vi "create s file from tdms of failed scan.vi"() -> ()   [LabVIEW 2020]
uses:
  Scan info_typdef.ctl
panel:
  in  "delete exising added channels":bool=TRUE
  out "TDMS path used":path
  out "appargs":string[](array[string])
  in  "append shot and bin #s":bool=TRUE
  out "device data Spreadsheet format":string[][](array[string])
  in  "TDMS path":path
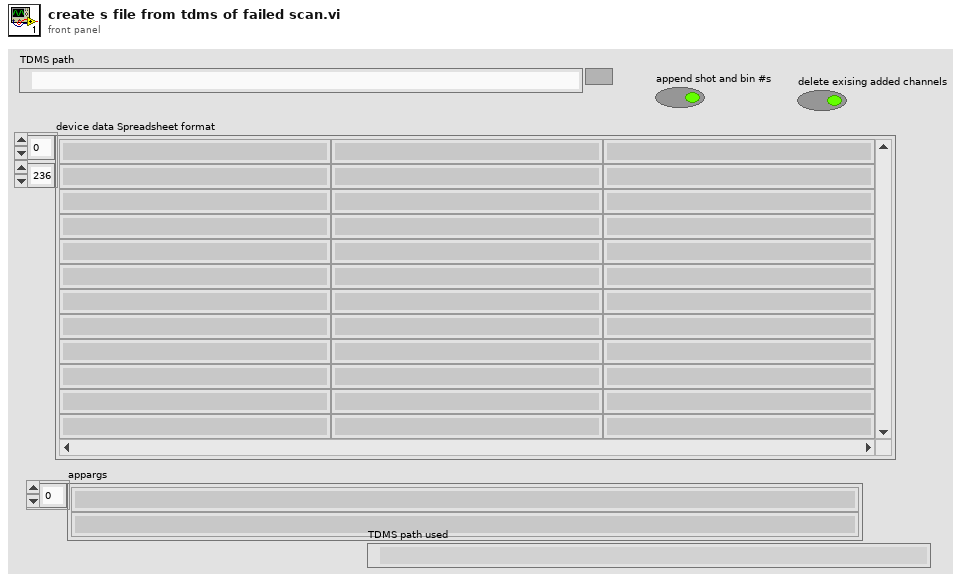
[diagram p1: front panel]
types:
  T1 = typedef "Scan info_typdef.ctl" = cluster{"# BG shots":i32, "Max Shot Number":i32, "Scan Number":i32}
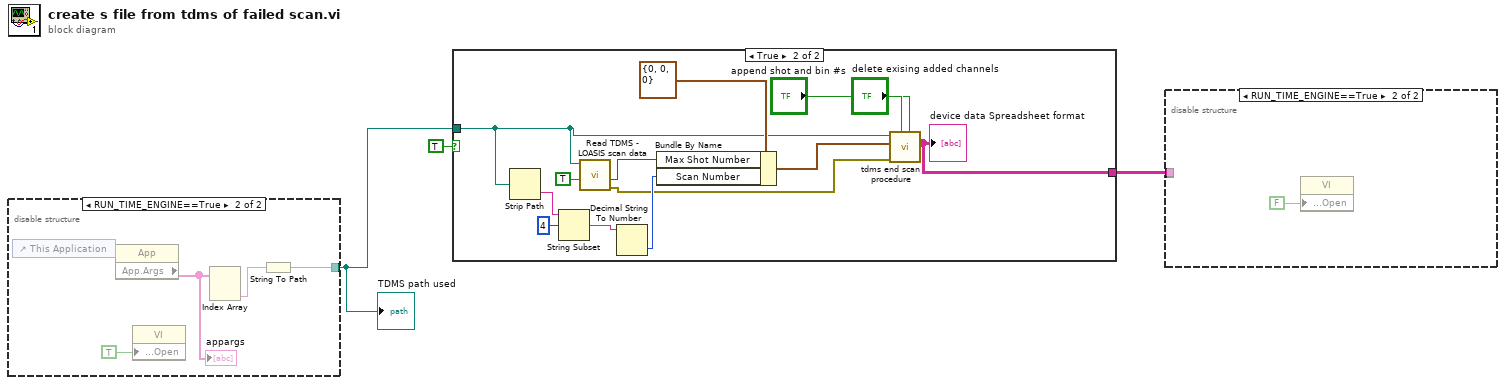
[diagram p0: block diagram]
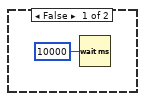
[diagram p3: hidden frame]
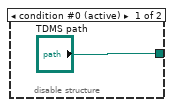
[diagram p4: hidden frame]
diagram:
  n1 = disable-structure shown="RUN_TIME_ENGINE==True" {
    disable-tunnel: ["TDMS path" w7] -> w3
    frame condition #0 (active) {
    }
    frame condition #1 {
      n2 = control-ref of="This Application"() -> (w9:refnum<vi>)
      n3 = property class="App"(reference=w9) -> ("App.Args"=w8:string[])  [unwired: 1 in, 2 out]
      "appargs" <- w8
      n4 = property class="VI"("Front Panel Window:Open"=TRUE) -> ()  [unwired: 2 in, 2 out]
      n5 = Index Array(array=w8) -> (element #2=w5:string)  [unwired: 2 in, 1 out]
      n6 = String To Path(string=w5) -> (path=w7:path)
    }
  }
  "TDMS path used" <- w3
  n7 = case shown="True" TRUE {
    tunnel: w3 -> [_ w14]
    tunnel: [_ w13] -> w1
    frame False {
      n8 = Wait (ms)(milliseconds to wait=u32 10000) -> ()  [unwired: 1 out]
    }
    frame True {
      n9 = Strip Path(path=w14) -> (name=w22:string)  [unwired: 1 out]
      n10 = String Subset(string=w22, offset (0)=4) -> (substring=w20:string)  [unwired: 1 in]
      n11 = call "Read TDMS - LOASIS scan data.vi"("UsingFilePath"=TRUE, "file path"=w14) -> ("error out"=w16:errorcluster, "max shot number"=w19:i32)  [unwired: 7 in, 1 out]
      n12 = Decimal String To Number(string=w20) -> (number=w18:i32)  [unwired: 2 in, 1 out]
      n13 = Bundle By Name(cluster=T1 {"# BG shots"=0, "Max Shot Number"=0, "Scan Number"=0} ("Scan info"), "Max Shot Number"=w19, "Scan Number"=w18) -> (w17:T1)
      n14 = call "tdms end scan procedure.vi"("delete exising added channels"="delete exising added channels", "append shot and bin #s"="append shot and bin #s", "error in (no error)"=w16, "Scan info"=w17, "TDMS path"=w14) -> ("device data Spreadsheet format"=w13:string[][])  [unwired: 4 in, 2 out]
      "device data Spreadsheet format" <- w13
    }
  }
  n15 = disable-structure shown="RUN_TIME_ENGINE==True" {
    disable-tunnel: [_ w24] -> _
    disable-tunnel: w1 -> [_ w24]
    frame condition #0 (active) {
    }
    frame condition #1 {
      n16 = property class="VI"("Front Panel Window:Open"=FALSE) -> ()  [unwired: 2 in, 2 out]
    }
  }
